vi "Starting.vi"(4 "Async Elements Queue":refnum<queue>, 6 "Actor Ref":refnum<vi>, 7 "Actor in":refnum<class "Actor.lvclass">, 9 "Attributes":refnum<class "Attributes.lvclass">, 10 "Refs":refnum<class "Refs.lvclass">) -> (0 "Error out":errorcluster, 2 "Address":refnum<data-value>, 5 "Actor out":refnum<class "Actor.lvclass">)   [LabVIEW 2025, in "jettl.lvlib" / "Queue Transport.lvlib"]
uses:
  Queue Transport.lvlib
  Actor/Actor.lvclass
  Attributes/Attributes.lvclass
  Refs/Refs.lvclass
  Msg/Msg.lvclass
  Async Elements/Async Elements.lvclass
  Queue Transport/Queue Transport.lvclass
  jettl.lvlib
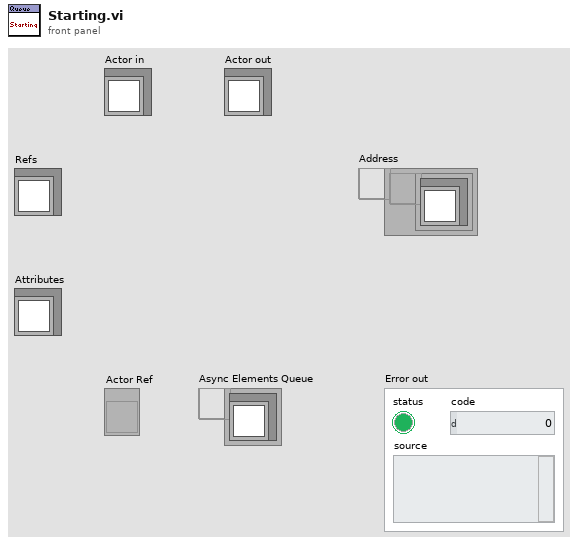
[diagram p1: front panel]
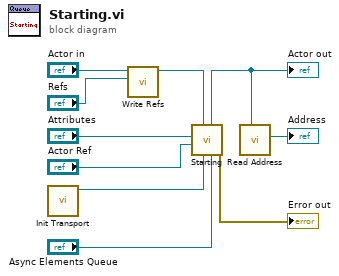
[diagram p0: block diagram]
diagram:
  n1 = call "Init Transport.vi"() -> ("Queue Transport out"=w4:refnum<class "Queue Transport.lvclass">)  [unwired: 11 in]
  n2 = call-dynamic "Write Refs.vi"("Refs"="Refs", "Actor in"="Actor in") -> ("Actor out"=w6:refnum<class "Actor.lvclass">)  [unwired: 9 in]
  n3 = call "Starting.vi"("Async Elements Queue"="Async Elements Queue", "Transport"=w4, "Actor in"=w6, "Actor Ref"="Actor Ref", "Attributes"="Attributes") -> ("Error out"=→"Error out":errorcluster, "Actor out"=w3:refnum<class "Actor.lvclass">)  [unwired: 5 in]
  "Actor out" <- w3
  n4 = call "Read Address.vi"("Actor"=w3) -> ("Address"=→"Address":refnum<data-value>)  [unwired: 10 in]
